vi "motorConsts.vi"(0 "Parameter":enum16{"P", "V", "T", "Kp", "Kd"}(ring)) -> (1 "Max":fxp<+/-,32,16>, 2 "Min":fxp<+/-,32,16>)   [LabVIEW 2019]
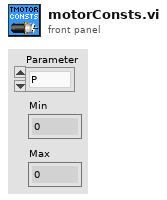
[diagram p1: front panel]
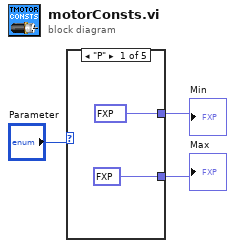
[diagram p0: block diagram]
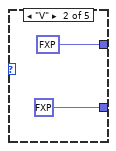
[diagram p2: hidden frame]
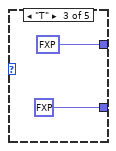
[diagram p3: hidden frame]
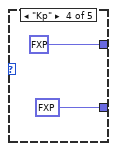
[diagram p4: hidden frame]
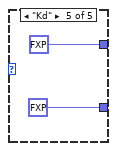
[diagram p5: hidden frame]
diagram:
  n1 = case shown="\"P\"" "Parameter" {
    tunnel: [fxp<+/-,9,8> -95.5 fxp<+/-,5,6> -30.0 fxp<+/-,5,6> -18.0 fxp<+,1,1> 0.0 fxp<+,1,1> 0.0] -> w2
    tunnel: [fxp<+,8,7> 95.5 fxp<+,4,5> 30.0 fxp<+,4,5> 18.0 fxp<+,7,9> 500.0 fxp<+,3,3> 5.0] -> w1
    frame "P" {
    }
    frame "V" {
    }
    frame "T" {
    }
    frame "Kp" {
    }
    frame "Kd" {
    }
  }
  "Min" <- w2
  "Max" <- w1
